vi "LWXPS_Example_FirmwareVersionGet.vi"() -> ()   [LabVIEW 2013]
panel:
  out "XPS Error String":string
  out "XPS Error code":i32
  out "Instrument Key OUT":string
  out "Error out":errorcluster caption="error out"
  out "Error code":i32
  out "XPS Controller Version":string
  in  "Instrument Key IN":string
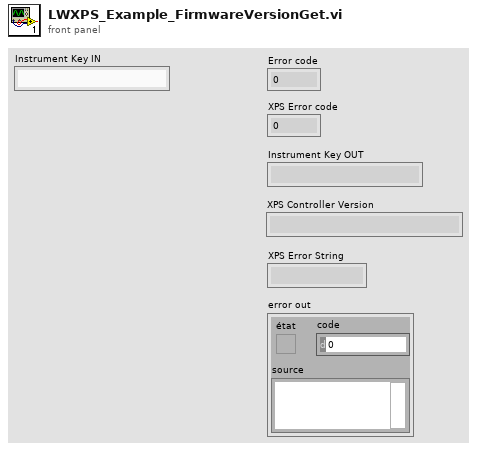
[diagram p1: front panel]
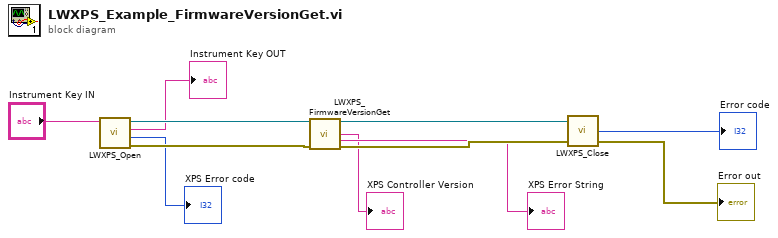
[diagram p0: block diagram]
diagram:
  n1 = call "LWXPS_Open.vi"("Instrument Key IN"="Instrument Key IN") -> ("error out"=w9:errorcluster, "Error code"=→"XPS Error code":i32, "Instrument Key OUT"=→"Instrument Key OUT":string, "CommandInterfaceXPS.XPS"=w11:refnum<k24>)  [unwired: 3 in]
  n2 = call "LWXPS_FirmwareVersionGet.vi"("CommandInterfaceXPS.XPS"=w11, "LabVIEW error IN"=w9) -> ("CommandInterfaceXPS.XPS"=w8:refnum<k24>, "XPS Controller Version"=→"XPS Controller Version":string, "XPS Error String"=→"XPS Error String":string, "LabVIEW error OUT"=w7:errorcluster)  [unwired: 9 in, 1 out]
  n3 = call "LWXPS_Close.vi"("error in (no error)"=w7, "XPS Reference"=w8) -> ("Error out"=→"Error out":errorcluster, "Error code"=→"Error code":i32)  [unwired: 2 in]
